vi "Set Zero Mode.vi"(8 "error in":errorcluster, 10 "Mode":u8 max=24 step=1, 11 "Neph in":refnum<class "Nephelometer.lvclass">) -> (0 "error out":errorcluster, 3 "Neph out":refnum<class "Nephelometer.lvclass">)   [LabVIEW 2014, in "Nephelometer.lvclass"]
doc: "Set the method used to zero the baseline drift using filtered air. The values are:\n* 0 = Manual\n* 1 = Normal mode in which zeroes are taken at regular intervals\n* 2-24 = aur cgio nide, similar to normal mode except that the last n values are averaged together"
uses:
  Nephelometer.lvclass
  Reusable/Session APIs/Serial/Serial Session.lvclass
  Nephelometer.lvclass/Nephelometer.ctl
  Accessors/Read Session Handle.vi
  <userlib>/_Session Fwk/Session - Root.lvclass
  Reusable/Session Log/System Log.lvclass
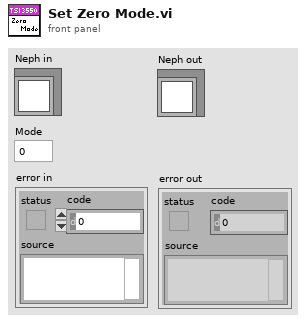
[diagram p1: front panel]
types:
  T1 = typedef "Session - Root.lvclass/Session Handle.ctl" = refnum<data-value>
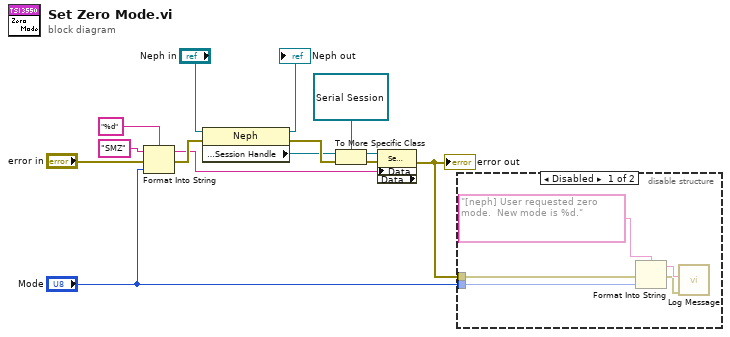
[diagram p0: block diagram]
diagram:
  n1 = Format Into String(format string="%d", initial string="SMZ", error in="error in", "Mode") -> (resulting string=w2:string, error out=w10:errorcluster)
  n2 = property class="Neph"(reference="Neph in", error in=w10) -> (reference out=→"Neph out":refnum<class "Nephelometer.lvclass">, error out=w7:errorcluster, "Accessors:Session Handle"=w3:T1)
  n3 = To More Specific Class(target class=refnum<data-value> refnum ("Session Handle"), reference=w3, error in=w7) -> (specific class reference=w5:refnum<data-value>, error out=w4:errorcluster)
  n4 = property class="Serial Session" props=["Data", "Data"](reference=w5, error in=w4, "Data"=w2) -> (error out=w1:errorcluster)  [unwired: 2 out]
  "error out" <- w1
  n5 = disable-structure shown="Disabled" {
    disable-tunnel: "Mode" -> [w19 _]
    disable-tunnel: w1 -> [w16 _]
    frame Disabled {
      n6 = Format Into String(format string="[neph] User requested zero mode.  New mode is %d.", error in=w16, w19) -> (resulting string=w17:string, error out=w15:errorcluster)  [unwired: 1 in]
      n7 = call "Log Message.vi"("error in"=w15, "MSG In"=w17) -> ()  [unwired: 8 in, 2 out]
    }
    frame Enabled {
    }
  }
